vi "Edit Config.vi"(8 "error in (no error)":errorcluster, 11 "NI Analog in":refnum<class "NI Analog.lvclass">) -> (0 "error out":errorcluster, 3 "NI Analog out":refnum<class "NI Analog.lvclass">)   [LabVIEW 2018, in "NI Analog.lvclass"]
doc: "NI Analog.lvclass:Edit Config.vi\n\nThis VI is used to edit the NI Analog configuration parameters.\n\nInstrument Communication Module Version 1.0\nJanuary, 2018 Original Code Consulting David Thomson\n www.originalcode.com"
uses:
  NI Analog.lvclass
  NI Analog Config.ctl
  NI Analog Channel Range.ctl
  Controls/ICM Class Editor State.ctl
  Controls/ICM Editor Command.ctl
  NI Analog.lvclass/NI Analog.ctl
panel:
  in  "Save":bool
  in  "Revert":bool
  in  "NI Analog Config":T1
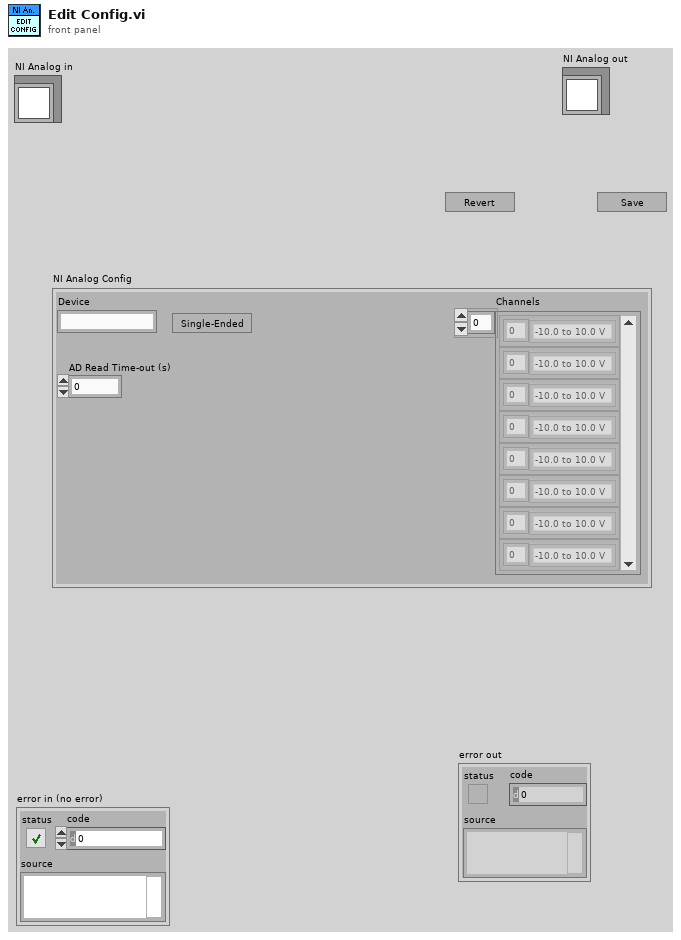
[diagram p1: front panel]
types:
  T1 = typedef "NI Analog Config.ctl" = cluster{"Device":string, "SE/Diff":bool, "Channels":cluster{"Channel":i32, "Range":T2}[], "AD Read Time-out (s)":dbl}
  T2 = typedef "NI Analog Channel Range.ctl" = enum16{"-10.0 to 10.0 V", "-5.0 to 5.0 V", "-2.0 to 2.0 V", "-1.0 to 1.0 V", "-0.5 to 0.5 V", "-0.2 to 0.2 V", "-0.1 to 0.1 V", "0 to 10 V", "0 to 5 V", "0 to 2 V", "0 to 1 V", "0 to 0.5 V", "0 to 0.2 V", "0 to 0.1 V"}
  T3 = typedef "ICM Editor Command.ctl" = enum16{"No-op", "Exit"}
  T4 = typedef "ICM Class Editor State.ctl" = enum16{"Init", "Wait", "Write", "Read", "Display", "Set Flashing", "Error", "Stop"}
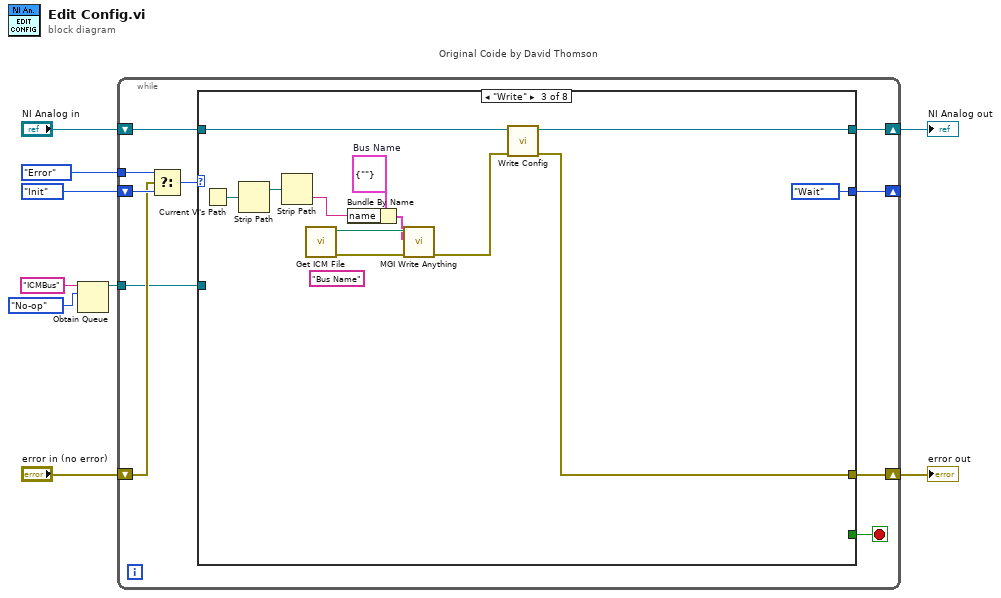
[diagram p0: block diagram]
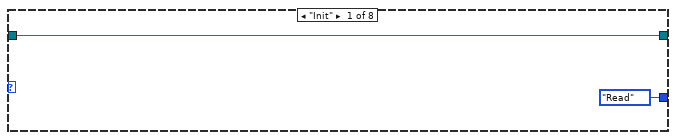
[diagram p2: hidden frame]
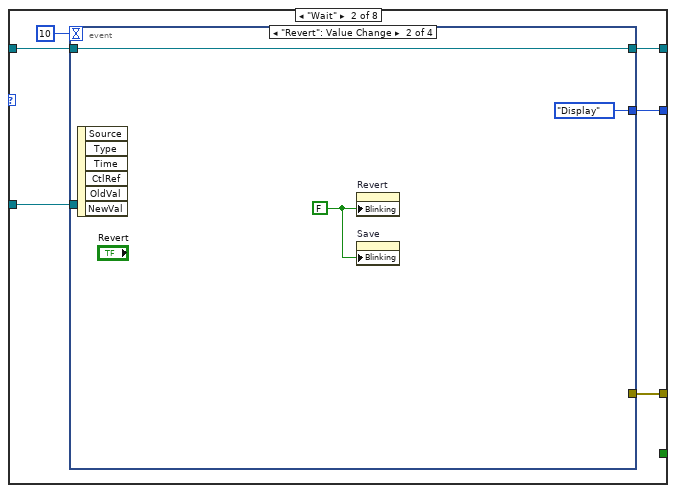
[diagram p3: hidden frame]
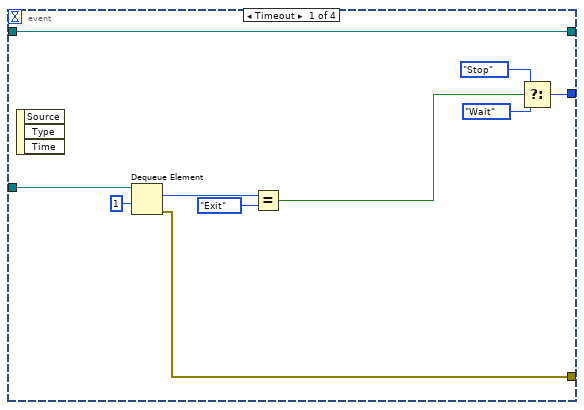
[diagram p4: hidden frame]
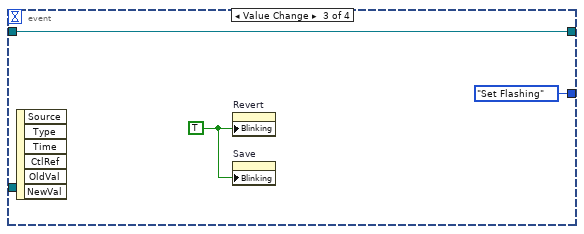
[diagram p5: hidden frame]
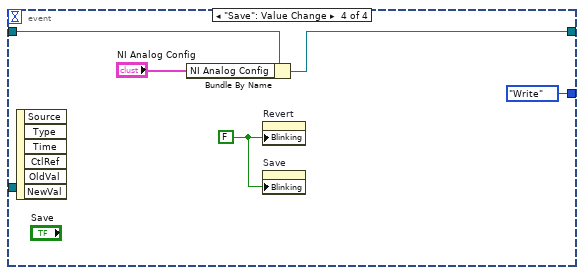
[diagram p6: hidden frame]
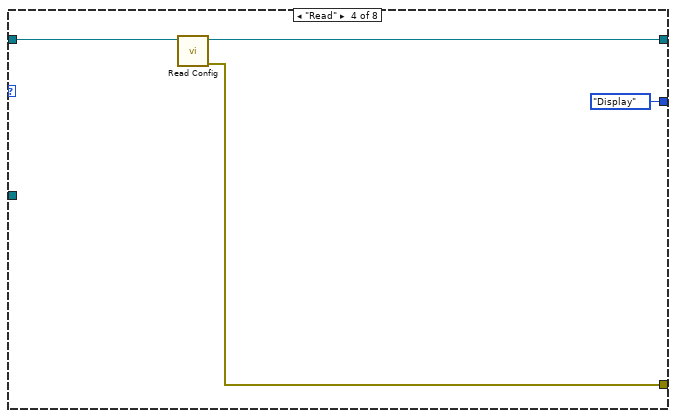
[diagram p7: hidden frame]
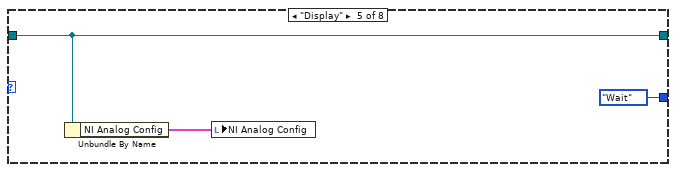
[diagram p8: hidden frame]
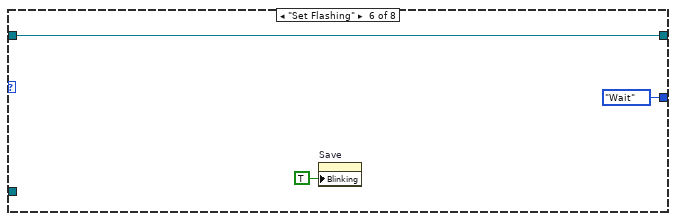
[diagram p9: hidden frame]
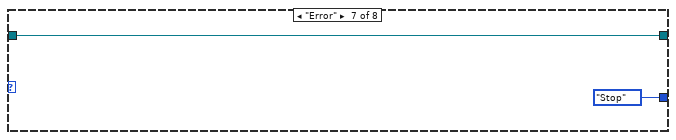
[diagram p10: hidden frame]
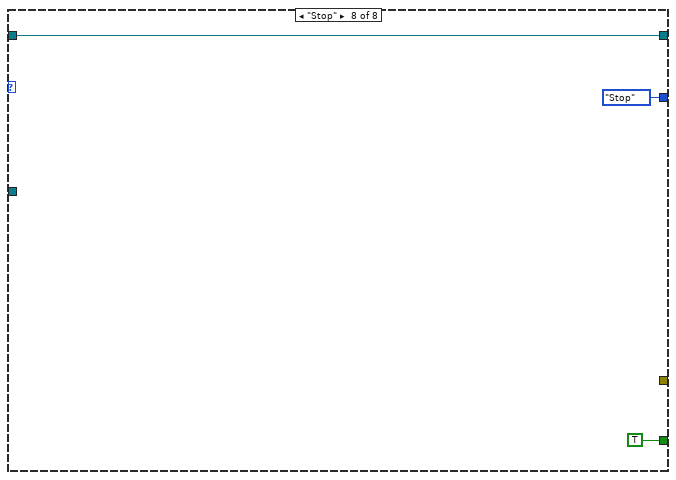
[diagram p11: hidden frame]
diagram:
  n1 = Obtain Queue(name (unnamed)="ICMBus", element data type=ICM_Editor_Command."No-op" ("Editor Command")) -> (queue out=w1:refnum<queue>)  [unwired: 3 in, 2 out]
  n2 = while "Original Coide by David Thomson" {
    shift-right: [w19] -> w8
    shift-left: "NI Analog in" -> [w18]
    shift-right: [w12] -> _
    shift-left: ICM_Class_Editor_State."Init" ("Config State") -> [w16]
    shift-right: [w11] -> w6
    shift-left: "error in (no error)" -> [w14]
    tunnel: ICM_Class_Editor_State."Error" ("Config State") -> [w13]
    tunnel: w1 -> [w10]
    stop <- w17 stop-if-true
    n3 = Select(t=w13, s=w14, f=w16) -> (s? t:f=w15:T4)
    n4 = case shown="\"Write\"" w15 {
      tunnel: [w20 w25 w58 w62 w67 w70 w72 w75] -> w19
      tunnel: w18 -> [w20 w24 w59 w64 w67 w70 w72 w75]
      tunnel: [_ _ _ _ _ _ _ TRUE] -> w17
      tunnel: [ICM_Class_Editor_State."Read" ("Config State") w26 ICM_Class_Editor_State."Wait" ("Config State") ICM_Class_Editor_State."Display" ("Config State") ICM_Class_Editor_State."Wait" ("Config State") ICM_Class_Editor_State."Wait" ("Config State") ICM_Class_Editor_State."Stop" ("Config State") ICM_Class_Editor_State."Stop" ("Config State")] -> w12
      tunnel: [_ w22 w57 w63 _ _ _ _] -> w11
      tunnel: w10 -> [_ w23 _ _ _ _ _ _]
      frame "Init" {
      }
      frame "Wait" {
        n5 = event shown="[1] \"Revert\": Value Change" {
          selector: _ -> [_ _ _ _]
          dyn-events: _ -> [_ _ _ _]
          timeout: 10 -> [_ _ _ _]
          tunnel: [w34 ICM_Class_Editor_State."Display" ("Config State") ICM_Class_Editor_State."Set Flashing" ("Config State") ICM_Class_Editor_State."Write" ("Config State")] -> w26
          tunnel: [w37 w39 w43 w45] -> w25
          tunnel: w24 -> [w37 w39 w43 w46]
          tunnel: w23 -> [w36 _ _ _]
          tunnel: [w28 _ _ _] -> w22
          event Timeout {
            n6 = event-data() -> ()  [unwired: 1 in, 3 out]
            n7 = Dequeue Element(queue=w36, timeout in ms (-1)=1) -> (element=w33:T3, error out=w28:errorcluster)  [unwired: 1 in, 2 out]
            n8 = Equal?(x=w33, y=ICM_Editor_Command."Exit") -> (x = y?=w31:bool)
            n9 = Select(t=ICM_Class_Editor_State."Stop" ("Config State"), s=w31, f=ICM_Class_Editor_State."Wait" ("Config State")) -> (s? t:f=w34:T4)
          }
          event "Revert": Value Change {
            w38 = FALSE ("Blinking")
            n10 = event-data() -> ()  [unwired: 1 in, 6 out]
            n11 = property on="Revert" class="Bool"("Blinking"=w38) -> ()  [unwired: 2 in, 2 out]
            n12 = property on="Save" class="Bool"("Blinking"=w38) -> ()  [unwired: 2 in, 2 out]
          }
          event Value Change {
            w41 = TRUE ("Blinking")
            n13 = event-data() -> ()  [unwired: 1 in, 6 out]
            n14 = property on="Revert" class="Bool"("Blinking"=w41) -> ()  [unwired: 2 in, 2 out]
            n15 = property on="Save" class="Bool"("Blinking"=w41) -> ()  [unwired: 2 in, 2 out]
          }
          event "Save": Value Change {
            w44 = FALSE ("Blinking")
            n16 = event-data() -> ()  [unwired: 1 in, 6 out]
            n17 = Bundle By Name(cluster=w46, "NI Analog Config"="NI Analog Config") -> (w45:refnum<class "NI Analog.lvclass">)
            n18 = property on="Revert" class="Bool"("Blinking"=w44) -> ()  [unwired: 2 in, 2 out]
            n19 = property on="Save" class="Bool"("Blinking"=w44) -> ()  [unwired: 2 in, 2 out]
          }
        }
      }
      frame "Write" {
        w51 = cluster{"name":string} {"name"=""}  # Bus Name
        (unwired) "Bus Name" ("Section Name (Name of \"Anything\")")
        n20 = Current VI's Path() -> (path=w56:path)
        n21 = Strip Path(path=w56) -> (stripped path=w55:path)  [unwired: 1 out]
        n22 = Strip Path(path=w55) -> (name=w50:string)  [unwired: 1 out]
        n23 = call "Get ICM File.vi"() -> ("error out"=w53:errorcluster, "ICM File"=w54:path)  [unwired: 10 in]
        n24 = Bundle By Name(cluster=w51, "name"=w50) -> (w49:cluster{"name":string})
        n25 = call <userlib>:"MGI Write Anything.vi"("Error In"=w53, "Anything"=w49, "Path (dialog)"=w54) -> ("Error Out"=w52:errorcluster)  [unwired: 6 in, 2 out]
        n26 = call-dynamic "Write Config.vi"("error in (no error)"=w52, "NI Analog in"=w59) -> ("error out"=w57:errorcluster, "NI Analog out"=w58:refnum<class "NI Analog.lvclass">)  [unwired: 8 in]
      }
      frame "Read" {
        n27 = call-dynamic "Read Config.vi"("NI Analog in"=w64) -> ("error out"=w63:errorcluster, "NI Analog out"=w62:refnum<class "NI Analog.lvclass">)  [unwired: 9 in]
      }
      frame "Display" {
        n28 = Unbundle By Name(w67) -> ("NI Analog Config"=w66:T1)
        n29 = local write "NI Analog Config"(w66) -> ()
      }
      frame "Set Flashing" {
        n30 = property on="Save" class="Bool"("Blinking"=TRUE) -> ()  [unwired: 2 in, 2 out]
      }
      frame "Error" {
      }
      frame "Stop" {
      }
    }
  }
  "error out" <- w6
  "NI Analog out" <- w8
